vi "DIAdem Lines To File Write.vi"(4 "error in (no error)":errorcluster, 5 "File Entries":string[](array[string]), 6 "File Path":path, 7 "File Name":string) -> (0 "error out":errorcluster, 3 "Result File Path":path)   [LabVIEW 2020]
doc: "Creates an ascii file using array string entries. An existing file will be overwritten."
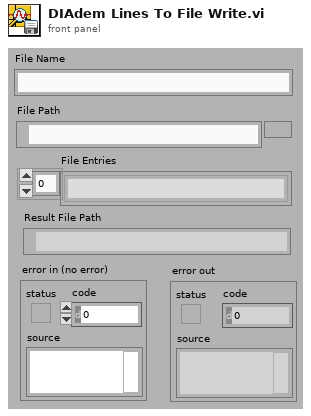
[diagram p1: front panel]
types:
  T1 = enum16{"open", "replace", "create", "open or create", "replace or create", "replace or create with confirmation"}
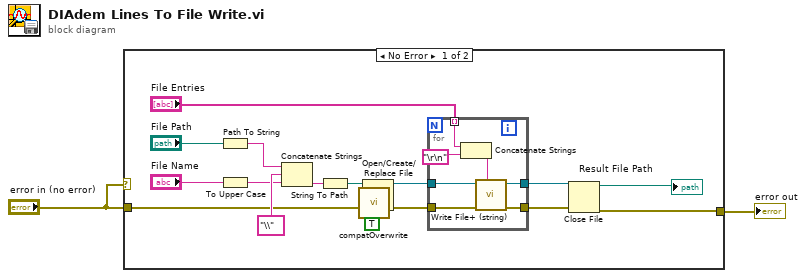
[diagram p0: block diagram]
diagram:
  n1 = case shown="No Error" "error in (no error)" {
    tunnel: "error in (no error)" -> [w12 w27]
    tunnel: [w14 w27] -> w1
    frame No Error {
      n2 = Path To String(path="File Path") -> (string=w16:string)
      n3 = To Upper Case(1:"File Name") -> (0:w4:string)
      n4 = Concatenate Strings(w16, "\\" ("Substring"), w4) -> (w18:string)
      n5 = String To Path(string=w18) -> (path=w13:path)
      n6 = call <vilib>:"compatOverwrite.vi"("overwrite (F)"=TRUE) -> ("overwrite?"=w3:T1)
      n7 = Open/Create/Replace File(file path (use dialog)=w13, error in=w12, operation (0:open)=w3) -> (refnum out=w7:refnum<file>, error out=w9:errorcluster)  [unwired: 3 in, 1 out]
      n8 = for {
        tunnel: w9 -> [w25]
        tunnel: [w24] -> w8
        tunnel: w7 -> [w23]
        tunnel: [w22] -> w6
        tunnel: "File Entries" -> [w20] mode=indexing
        n9 = Concatenate Strings(w20, "\r\n") -> (w21:string)
        n10 = call <vilib>:"Write File+ (string).vi"("string"=w21, "error in (no error)"=w25, "refnum"=w23) -> ("error out"=w24:errorcluster, "dup refnum"=w22:refnum<file>)  [unwired: 4 in, 1 out]
      }
      n11 = Close File(refnum=w6, error in=w8) -> (path=→"Result File Path":path, error out=w14:errorcluster)
    }
    frame Error {
    }
  }
  "error out" <- w1
